vi "Settings Dialog.vi"(8 "error in (no error)":errorcluster caption="错误输入（无错误）", 11 "Settings in":T6={"DAQ Configuration"={"hDevice"=0, "DevNum"=0, "Configuration Parameter"=[], "READ_MAX_LEN"=10146, "DO"=[]}, "DSP Configuration"={"Sampling Frequency"=0.0, "filter type"=enum."Lowpass", "RF Filter Low Frequency"=0.0, "RF Filter High Frequency"=0.0, "RF Filter Taps"=0, "window"=0, "RF window parameter"=nan, "filter type 2"=enum."Lowpass", "Demodulated Filter Low Frequency"=0.0, "Demodulated Filter HighFrequency"=0.0, "Demodulated Filter Order"=0, "SPAN"=10092, "Logarithmic Base"=2.0, "Noise path"="", "Work position parameter"=[]}, "Biometry Configuration"={"Interference Width"=0, "Interference Threshold"=0.0, "Cornea Len Division"=0, "Correction Data 1st Path"="", "1st_Start_Position"=2.0, "Correction Data 2nd Path"="", "2nd_Start_Position"=0.0, "Index Corneal"=0.0, "Index Water"=0.0, "Index Len"=2.0, "Working Position"={"FirstStart"=9600, "FirstEnd"=0, "SecondStart"=0, "SecondEnd"=0}}} caption="设置" {"DSP Configuration"."window" items=["Rectangle"=0, "Hanning"=1, "Hamming"=2, "Blackman-Harris"=3, "Exact Blackman"=4, "Blackman"=5, "Flat Top"=6, "4 Term B-Harris "=7, "7 Term B-Harris"=8, "Low Sidelobe"=9, "Blackman Nuttall"=11, "Triangle"=30, "Bartlett-Hanning"=31, "Bohman"=32, "Parzen"=33, "Welch"=34, "Kaiser"=60, "Dolph-Chebyshev"=61, "Gaussian"=62]}) -> (0 "error out":errorcluster caption="错误输出", 1 "Cancelled?":bool=TRUE caption="取消？", 2 "UI Refresh Needed?":bool caption="需要刷新UI？", 3 "Settings out":T6={"DAQ Configuration"={"hDevice"=0, "DevNum"=0, "Configuration Parameter"=[], "READ_MAX_LEN"=10146, "DO"=[]}, "DSP Configuration"={"Sampling Frequency"=0.0, "filter type"=enum."Lowpass", "RF Filter Low Frequency"=0.0, "RF Filter High Frequency"=0.0, "RF Filter Taps"=0, "window"=0, "RF window parameter"=nan, "filter type 2"=enum."Lowpass", "Demodulated Filter Low Frequency"=0.0, "Demodulated Filter HighFrequency"=0.0, "Demodulated Filter Order"=0, "SPAN"=10092, "Logarithmic Base"=2.0, "Noise path"="", "Work position parameter"=[]}, "Biometry Configuration"={"Interference Width"=0, "Interference Threshold"=0.0, "Cornea Len Division"=0, "Correction Data 1st Path"="", "1st_Start_Position"=2.0, "Correction Data 2nd Path"="", "2nd_Start_Position"=0.0, "Index Corneal"=0.0, "Index Water"=0.0, "Index Len"=2.0, "Working Position"={"FirstStart"=9600, "FirstEnd"=0, "SecondStart"=0, "SecondEnd"=0}}} caption="设置" {"DSP Configuration"."window" items=["Rectangle"=0, "Hanning"=1, "Hamming"=2, "Blackman-Harris"=3, "Exact Blackman"=4, "Blackman"=5, "Flat Top"=6, "4 Term B-Harris "=7, "7 Term B-Harris"=8, "Low Sidelobe"=9, "Blackman Nuttall"=11, "Triangle"=30, "Bartlett-Hanning"=31, "Bohman"=32, "Parzen"=33, "Welch"=34, "Kaiser"=60, "Dolph-Chebyshev"=61, "Gaussian"=62]})   [LabVIEW 2015, in "Settings.lvlib"]
doc: "用于选择用户设置的对话框。"
uses:
  Settings.lvlib
  Settings.ctl
  Sub VIs/DAQ/DAQ Configuration.ctl
  Sub VIs/Digital Signal Processing/Support/DSP Configuration.ctl
  <vilib>/Analysis/3filter.llb/Filter Passband Type.ctl
  <vilib>/Analysis/4window.llb/windowTd.ctl
  Sub VIs/Boimetry Processing/Controls/Biometry Configuration.ctl
  <vilib>/Utility/xml.llb/Write to XML File(string).vi
  Sub VIs/DAQ/DAQ.lvlib
  Sub VIs/Boimetry Processing/Boimetry Processing.lvlib
  <vilib>/Analysis/NI_AALBase.lvlib
  <vilib>/Analysis/NI_AALPro.lvlib
  Sub VIs/Digital Signal Processing/Digital Signal Processing.lvlib
panel:
  in  "Biometry Configuration":T1
  in  "DSP Configuration":T2={"Sampling Frequency"=0.0, "filter type"=enum."Lowpass", "RF Filter Low Frequency"=0.0, "RF Filter High Frequency"=0.0, "RF Filter Taps"=0, "window"=0, "RF window parameter"=nan, "filter type 2"=enum."Lowpass", "Demodulated Filter Low Frequency"=0.0, "Demodulated Filter HighFrequency"=0.0, "Demodulated Filter Order"=0, "SPAN"=0, "Logarithmic Base"=0.0, "Noise path"="", "Work position parameter"=[]} {"window" items=["Rectangle"=0, "Hanning"=1, "Hamming"=2, "Blackman-Harris"=3, "Exact Blackman"=4, "Blackman"=5, "Flat Top"=6, "4 Term B-Harris "=7, "7 Term B-Harris"=8, "Low Sidelobe"=9, "Blackman Nuttall"=11, "Triangle"=30, "Bartlett-Hanning"=31, "Bohman"=32, "Parzen"=33, "Welch"=34, "Kaiser"=60, "Dolph-Chebyshev"=61, "Gaussian"=62]}
  in  "DAQ Configuration":T5
  in  "Cancel Button":bool caption="取消按钮"
  in  "OK Button":bool caption="确定按钮"
  # "设置"
  # "对话框不可见部分（用于连线板）"
  # "lChCnt"
  # "lSelClk"
  # "lClkDiv"
  # "TriggerMode"
  # "TriggerSource"
  # "TriggerDelay"
  # "TriggerLength"
  # "TriggerLevel"
  # "lSelDataSrc"
  # "lExtTrigDelay"
  # "lADFmt"
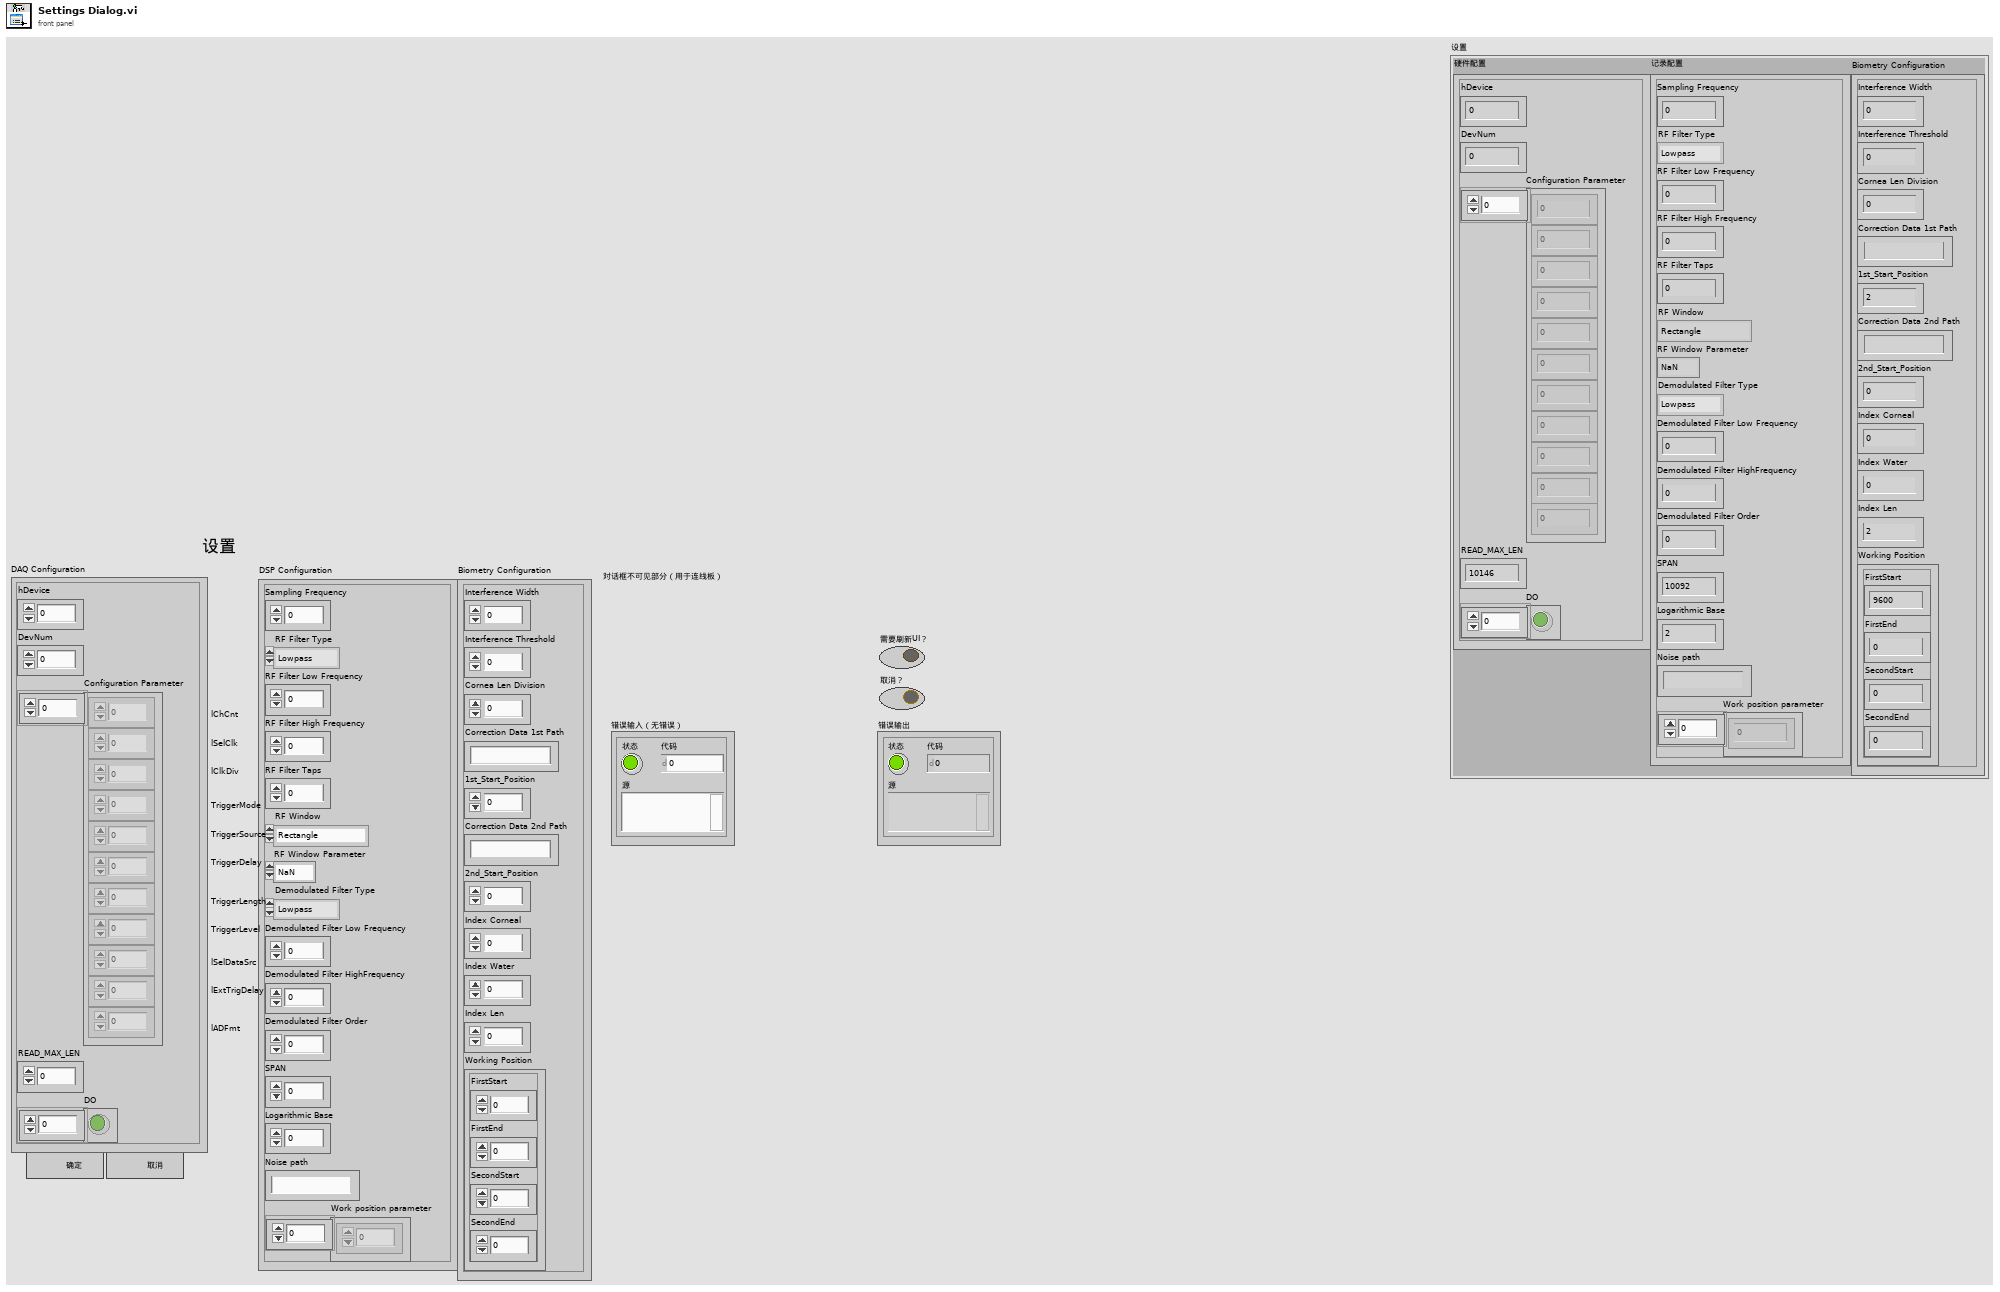
[diagram p1: front panel]
types:
  T1 = typedef "Boimetry Processing.lvlib/Biometry Configuration.ctl" = cluster{"Interference Width":i32, "Interference Threshold":dbl, "Cornea Len Division":i32, "Correction Data 1st Path":string, "1st_Start_Position":dbl, "Correction Data 2nd Path":string, "2nd_Start_Position":dbl, "Index Corneal":dbl, "Index Water":dbl, "Index Len":dbl, "Working Position":cluster{"FirstStart":i32, "FirstEnd":i32, "SecondStart":i32, "SecondEnd":i32}}
  T2 = typedef "Digital Signal Processing.lvlib/DSP Configuration.ctl" = cluster{"Sampling Frequency":dbl, "filter type":T3, "RF Filter Low Frequency":dbl, "RF Filter High Frequency":dbl, "RF Filter Taps":i32, "window":T4, "RF window parameter":dbl, "filter type 2":T3, "Demodulated Filter Low Frequency":dbl, "Demodulated Filter HighFrequency":dbl, "Demodulated Filter Order":i32, "SPAN":i32, "Logarithmic Base":dbl, "Noise path":string, "Work position parameter":i32[]}
  T3 = typedef "NI_AALBase.lvlib/Filter Passband Type.ctl" = enum32{"Lowpass", "Highpass", "Bandpass", "Bandstop"}
  T4 = typedef "NI_AALPro.lvlib/windowTd.ctl" = u32
  T5 = typedef "DAQ.lvlib/DAQ Configuration.ctl" = cluster{"hDevice":i32, "DevNum":u8, "Configuration Parameter":i32[], "READ_MAX_LEN":i32, "DO":bool[]}
  T6 = typedef "Settings.lvlib/Settings.ctl" = cluster{"DAQ Configuration":T5, "DSP Configuration":T2, "Biometry Configuration":T1}
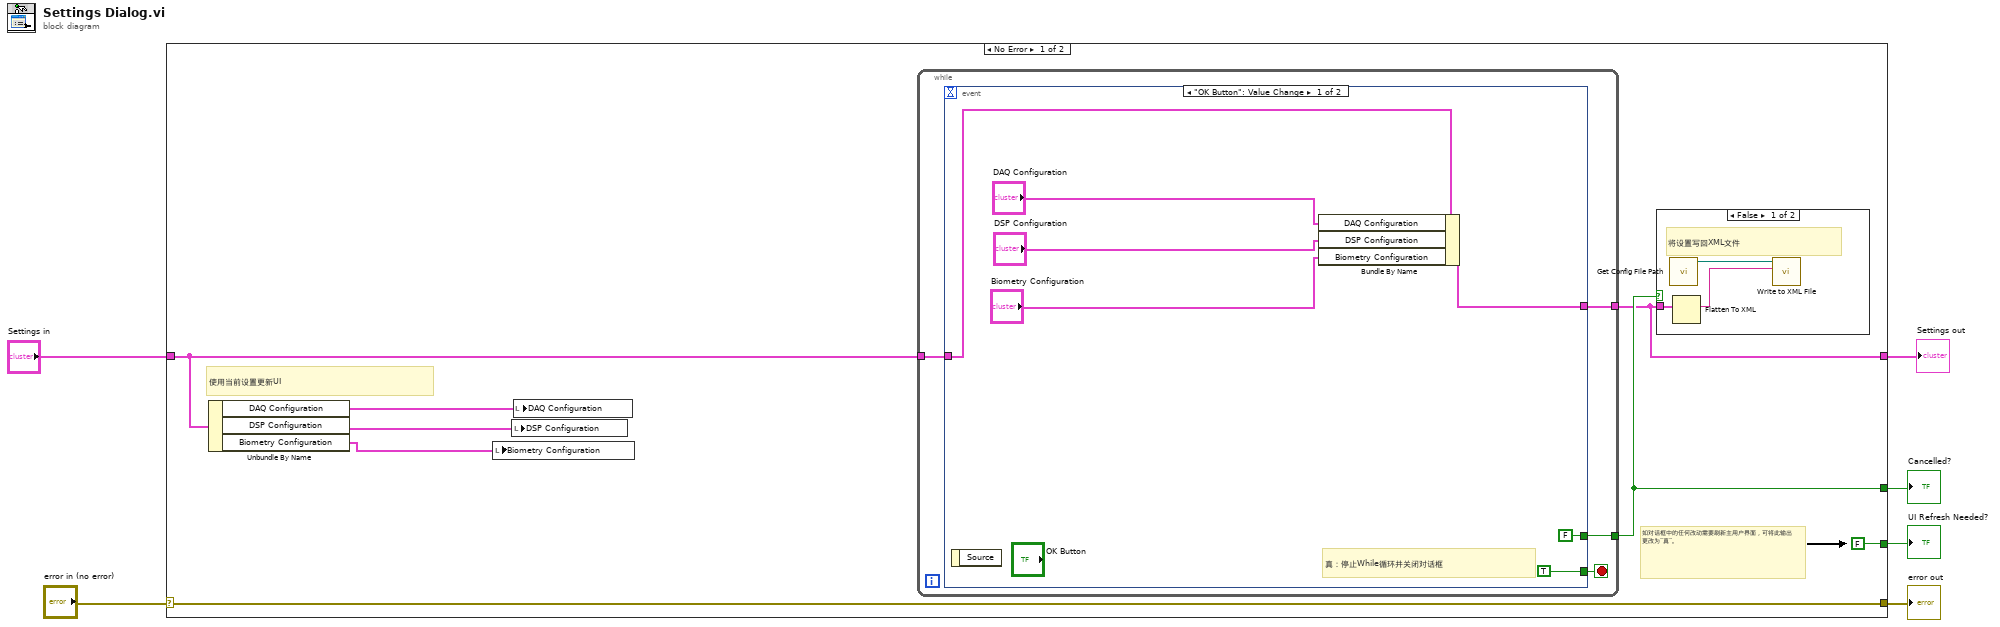
[diagram p0: block diagram]
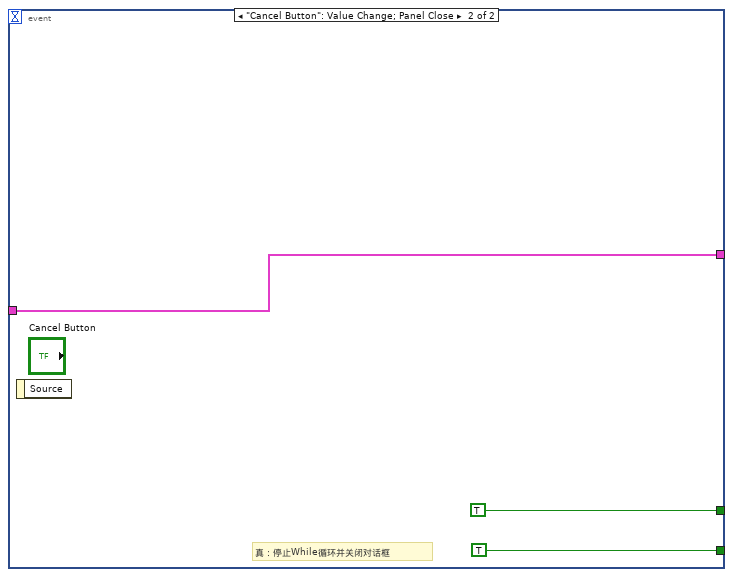
[diagram p2: hidden frame]
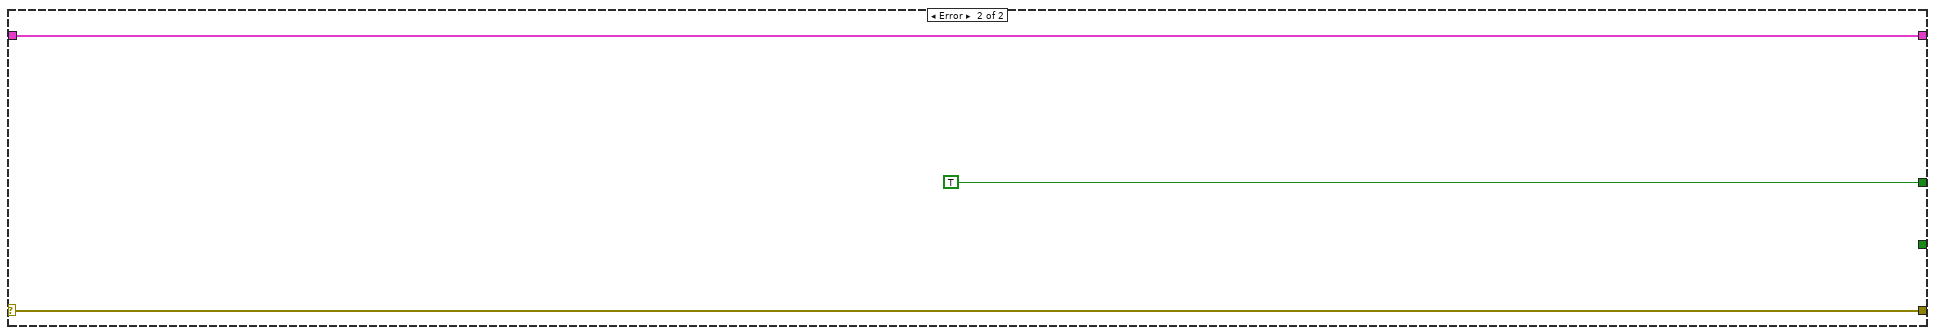
[diagram p4: hidden frame]
diagram:
  n1 = case shown="No Error" "error in (no error)" {
    selector: "error in (no error)" -> [w14 w34]
    tunnel: [w14 w34] -> w6
    tunnel: "Settings in" -> [w10 w33]
    tunnel: [w11 w33] -> w1
    tunnel: [FALSE ("UI Refresh Needed?") _] -> w5
    tunnel: [w12 TRUE ("UI Refresh Needed?")] -> w4
    frame No Error {
      # "使用当前设置更新UI"
      # "如对话框中的任何改动需要刷新主用户界面，可将此输出更改为“真”。"
      n2 = Unbundle By Name(w10) -> ("DAQ Configuration"=w9:T5, "DSP Configuration"=w8:T2, "Biometry Configuration"=w7:T1)
      n3 = local write "Biometry Configuration"(w7) -> ()
      n4 = local write "DSP Configuration"(w8) -> ()
      n5 = local write "DAQ Configuration"(w9) -> ()
      n6 = while {
        tunnel: [w18] -> w12
        tunnel: [w17] -> w11
        tunnel: w10 -> [w16]
        stop <- w15 stop-if-true
        n7 = event shown="[0] \"OK Button\": Value Change" {
          selector: _ -> [_ _]
          dyn-events: _ -> [_ _]
          timeout: _ -> [_ _]
          tunnel: [w23 w28] -> w17
          tunnel: w16 -> [w22 w28]
          tunnel: [FALSE ("UI Refresh Needed?") TRUE ("UI Refresh Needed?")] -> w18
          tunnel: [TRUE TRUE] -> w15
          event "OK Button": Value Change {
            # "真：停止While循环并关闭对话框"
            n8 = event-data() -> ()  [unwired: 1 in, 1 out]
            n9 = Bundle By Name(cluster=w22, "DAQ Configuration"="DAQ Configuration", "DSP Configuration"="DSP Configuration", "Biometry Configuration"="Biometry Configuration") -> (w23:T6)
          }
          event "Cancel Button": Value Change; Panel Close {
            # "真：停止While循环并关闭对话框"
            n10 = event-data() -> ()  [unwired: 1 in, 1 out]
          }
        }
      }
      n11 = case shown="False" w12 {
        tunnel: w11 -> [w30 _]
        frame False {
          # "将设置写回XML文件"
          n12 = call "Get Config File Path.vi"() -> ("XML File Path"=w31:path)  [unwired: 10 in, 1 out]
          n13 = Flatten To XML(anything=w30) -> (xml string=w29:string)
          n14 = call-poly <vilib>:"Write to XML File.vi"("XML Input"=w29, "XML File Path"=w31) -> ()  [unwired: 7 in, 3 out]
        }
        frame True {
        }
      }
    }
    frame Error {
    }
  }
  "UI Refresh Needed?" <- w5
  "error out" <- w6
  "Cancelled?" <- w4
  "Settings out" <- w1
